vi "PmacCommGlobal.vi"() -> ()   [LabVIEW 2020]
doc: "This VI is a Global copy of the PmacCommGlobal.ctl cluster used by servel PmacComm VIs for error reporting and logging purposes."
panel:
  out "Pmac Comm Global Cluster":T1 {"Num Commands i32" min=0}
  # "->"
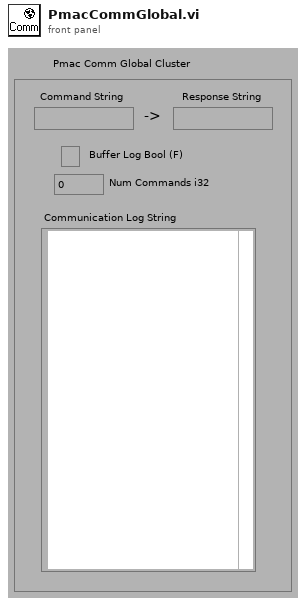
[diagram p1: front panel]
types:
  T1 = cluster{"Command String":string, "Response String":string, "Communication Log String":string, "Num Commands i32":i32, "Buffer Log Bool (F)":bool}
diagram:
